vi "Format Value (1D).vi"(1 "Array (DBL)":dbl[](array[numeric]), 2 "format string":string, 3 "string (\"\")":string) -> (0 "String Array":string[](array[string]))   [LabVIEW 2020]
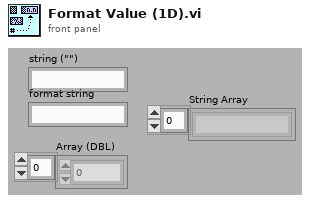
[diagram p1: front panel]
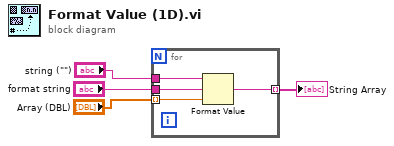
[diagram p0: block diagram]
diagram:
  n1 = for {
    tunnel: "Array (DBL)" -> [w8] mode=indexing
    tunnel: "format string" -> [w7]
    tunnel: [w6] -> w4 mode=indexing
    tunnel: "string (\"\")" -> [w5]
    n2 = Format Value(string ("")=w5, format string=w7, value (0)=w8) -> (output string=w6:string)
  }
  "String Array" <- w4
